vi "Teleop.vi"(10 "Match Info":T1={"Autonomous Elapsed Seconds"=0.0, "TeleOp Elapsed Seconds"=0.0, "Disabled Elapsed Seconds"=0.0, "Visited Autonomous"=FALSE, "Visited TeleOp"=FALSE, "Visited Disabled"=FALSE, "Autonomous Settings"={"Autonomous Style"=enum."Independent", "VI Refnum"=refnum}}, 11 "Call Context":T2) -> ()   [LabVIEW 2020]
doc: "This VI is called for each TeleOp packet received from the DS where the robot is not disabled. It is often used to read from the joysticks and update I/O or to update setpoints for timed control loops. It should complete and return within 20 milliseconds or it may miss DS packets."
uses:
  <vilib>/Rock Robotics/WPI/DriverStation/WPI_DriverStationDerivedRobotMode.ctl
  <vilib>/Rock Robotics/WPI/DriverStation/WPI_DriverStationMatch Info.ctl
  <vilib>/Rock Robotics/WPI/ThirdParty/Phoenix-LabVIEW/Motor Controller/Controls/CTRE_Phoenix_MotorControl_ControlMode.ctl
  <vilib>/Rock Robotics/WPI/Solenoid/WPI_SolenoidValue.ctl
  <vilib>/Rock Robotics/WPI/Utilities/WPI_GetSetVariantRefNum.vi
  <vilib>/Rock Robotics/Network Tables/NT Write Boolean Array.vi
  <vilib>/Rock Robotics/Network Tables/NT Write Numeric Array.vi
  <vilib>/Rock Robotics/Network Tables/NT Read Boolean.vi
  <vilib>/Rock Robotics/Network Tables/NT Read Number.vi
  Robot Global Data.vi
  <vilib>/Rock Robotics/WPI/ThirdParty/Phoenix-LabVIEW/Motor Controller/Get/CTRE_Phoenix_MotorController_GetSelectedSensorData.vi
  <vilib>/Rock Robotics/WPI/Solenoid/WPI_SolenoidSetEnum.vi
  <vilib>/Rock Robotics/WPI/ThirdParty/Phoenix-LabVIEW/Pigeon IMU/CTRE_PigeonIMU_GetAccumGyro.vi
panel:
  out "Left Motor Encoder":i32
  out "AccumGyro":cluster{"X":dbl, "Y":dbl, "Z":dbl}
  out "Intake Output":dbl
  out "Sample Slider 0":dbl(slide) scale=0.0..5.0
  out "Sample Boolean 1":bool
  out "Sample Boolean 0":bool
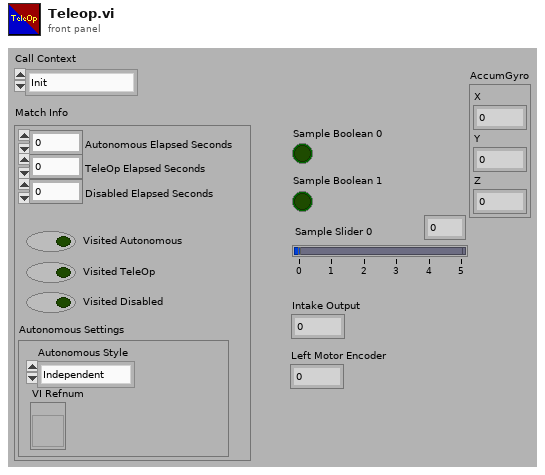
[diagram p1: front panel]
types:
  T1 = typedef "WPI_DriverStationMatch Info.ctl" = cluster{"Autonomous Elapsed Seconds":dbl, "TeleOp Elapsed Seconds":dbl, "Disabled Elapsed Seconds":dbl, "Visited Autonomous":bool, "Visited TeleOp":bool, "Visited Disabled":bool, "Autonomous Settings":cluster{"Autonomous Style":enum16{"Iterative", "Independent"}, "VI Refnum":refnum<vi>}}
  T2 = typedef "WPI_DriverStationDerivedRobotMode.ctl" = enum16{"Init", "Execute", "Stop"}
  T3 = typedef "WPI_SolenoidValue.ctl" = enum16{"Off", "On", "Forward", "Reverse"}
  T4 = typedef "CTRE_Phoenix_MotorControl_ControlMode.ctl" = u16
  T5 = typedef "WPI_JoystickDevRef.ctl" = cluster{"Device":T6}
  T6 = typedef "WPI_JoystickDeviceEnum.ctl" = enum16{"USB 0", "USB 1", "USB 2", "USB 3", "USB 4", "USB 5"}
  T7 = typedef "CTRE_PigeonIMU_DeviceRef.ctl" = cluster{"DeviceStatus":errorcluster, "Device Number":u8, "Type":T8, "Device ID":u32, "Handle":u64, "UsageFrame":u32, "Library Path":path}
  T8 = typedef "CTRE_PigeonIMU_ConnectionType.ctl" = u32
  T9 = typedef "WPI_MotorControlDeviceRef.ctl" = cluster{"DeviceStatus":errorcluster, "Type":T10, "PWM":cluster{"PWM Channel":T11, "DeadBand":T12}, "CAN":cluster{"Device Number":u8, "SetOutput VI Ref":variant, "GetOutput VI Ref":variant, "Enable VI Ref":variant, "Disable VI Ref":variant, "Data":variant}, "Invert":bool, "DIO PWM":cluster{"PWM \"Enable\" Channel":T11, "DIOChannel":T13, "PWM Rate":dbl}}
  T10 = typedef "WPI_MotorControlType.ctl" = enum16{"PWM", "CAN", "DIO PWM"}
  T11 = typedef "FPGA_DIOPWMChannel.ctl" = enum8{"PWM 0", "PWM 1", "PWM 2", "PWM 3", "PWM 4", "PWM 5", "PWM 6", "PWM 7", "PWM 8", "PWM 9", "PWM MXP 0", "PWM MXP 1", "PWM MXP 2", "PWM MXP 3", "PWM MXP 4", "PWM MXP 5", "PWM MXP 6", "PWM MXP 7", "PWM MXP 8", "PWM MXP 9", "Invalid"}
  T12 = typedef "WPI_PWMDeadband.ctl" = cluster{"Name":string, "maxPositivePwm":i32, "minPositivePwm":i32, "centerPwm":i32, "maxNegativePwm":i32, "minNegativePwm":i32, "angularRange":u16}
  T13 = typedef "FPGA_DIOChannel.ctl" = enum8{"DIO 0", "DIO 1", "DIO 2", "DIO 3", "DIO 4", "DIO 5", "DIO 6", "DIO 7", "DIO 8", "DIO 9", "DIO MXP 0", "DIO MXP 1", "DIO MXP 2", "DIO MXP 3", "DIO MXP 4", "DIO MXP 5", "DIO MXP 6", "DIO MXP 7", "DIO MXP 8", "DIO MXP 9", "DIO MXP 10", "DIO MXP 11", "DIO MXP 12", "DIO MXP 13", "DIO MXP 14", "DIO MXP 15", "SPI Port CS1", "SPI Port CS2", "SPI Port CS3", "SPI Port MISO", "SPI Port MOSI", "Invalid"}
  T14 = typedef "WPI_RobotDriveDevRef.ctl" = cluster{"DevStatus":errorcluster, "Motors[]":T9[], "Square Inputs":bool, "Max Output":dbl}
  T15 = typedef "WPI_SolenoidDevRef.ctl" = cluster{"DevStatus":errorcluster, "Pneumatics Control Module":u8, "Forward Solenoid Channel":T16, "Reverse Solenoid Channel":T16}
  T16 = typedef "WPI_SolenoidChannel.ctl" = enum8{"Solenoid 0", "Solenoid 1", "Solenoid 2", "Solenoid 3", "Solenoid 4", "Solenoid 5", "Solenoid 6", "Solenoid 7", "Solenoid 8", "Solenoid 9", "Solenoid 10", "Solenoid 11", "Solenoid 12", "Solenoid 13", "Solenoid 14", "Solenoid 15", "Invalid"}
  T17 = typedef "WPI_SwitchDevRef.ctl" = cluster{"DevStatus":errorcluster, "DIO Channel":T13, "CntIndex":T18, "Normally Closed":bool}
  T18 = typedef "FPGA_CounterCtrSystemIndex.ctl" = enum8{"Ctr 0", "Ctr 1", "Ctr 2", "Ctr 3", "Ctr 4", "Ctr 5", "Ctr 6", "Ctr 7", "Invalid"}
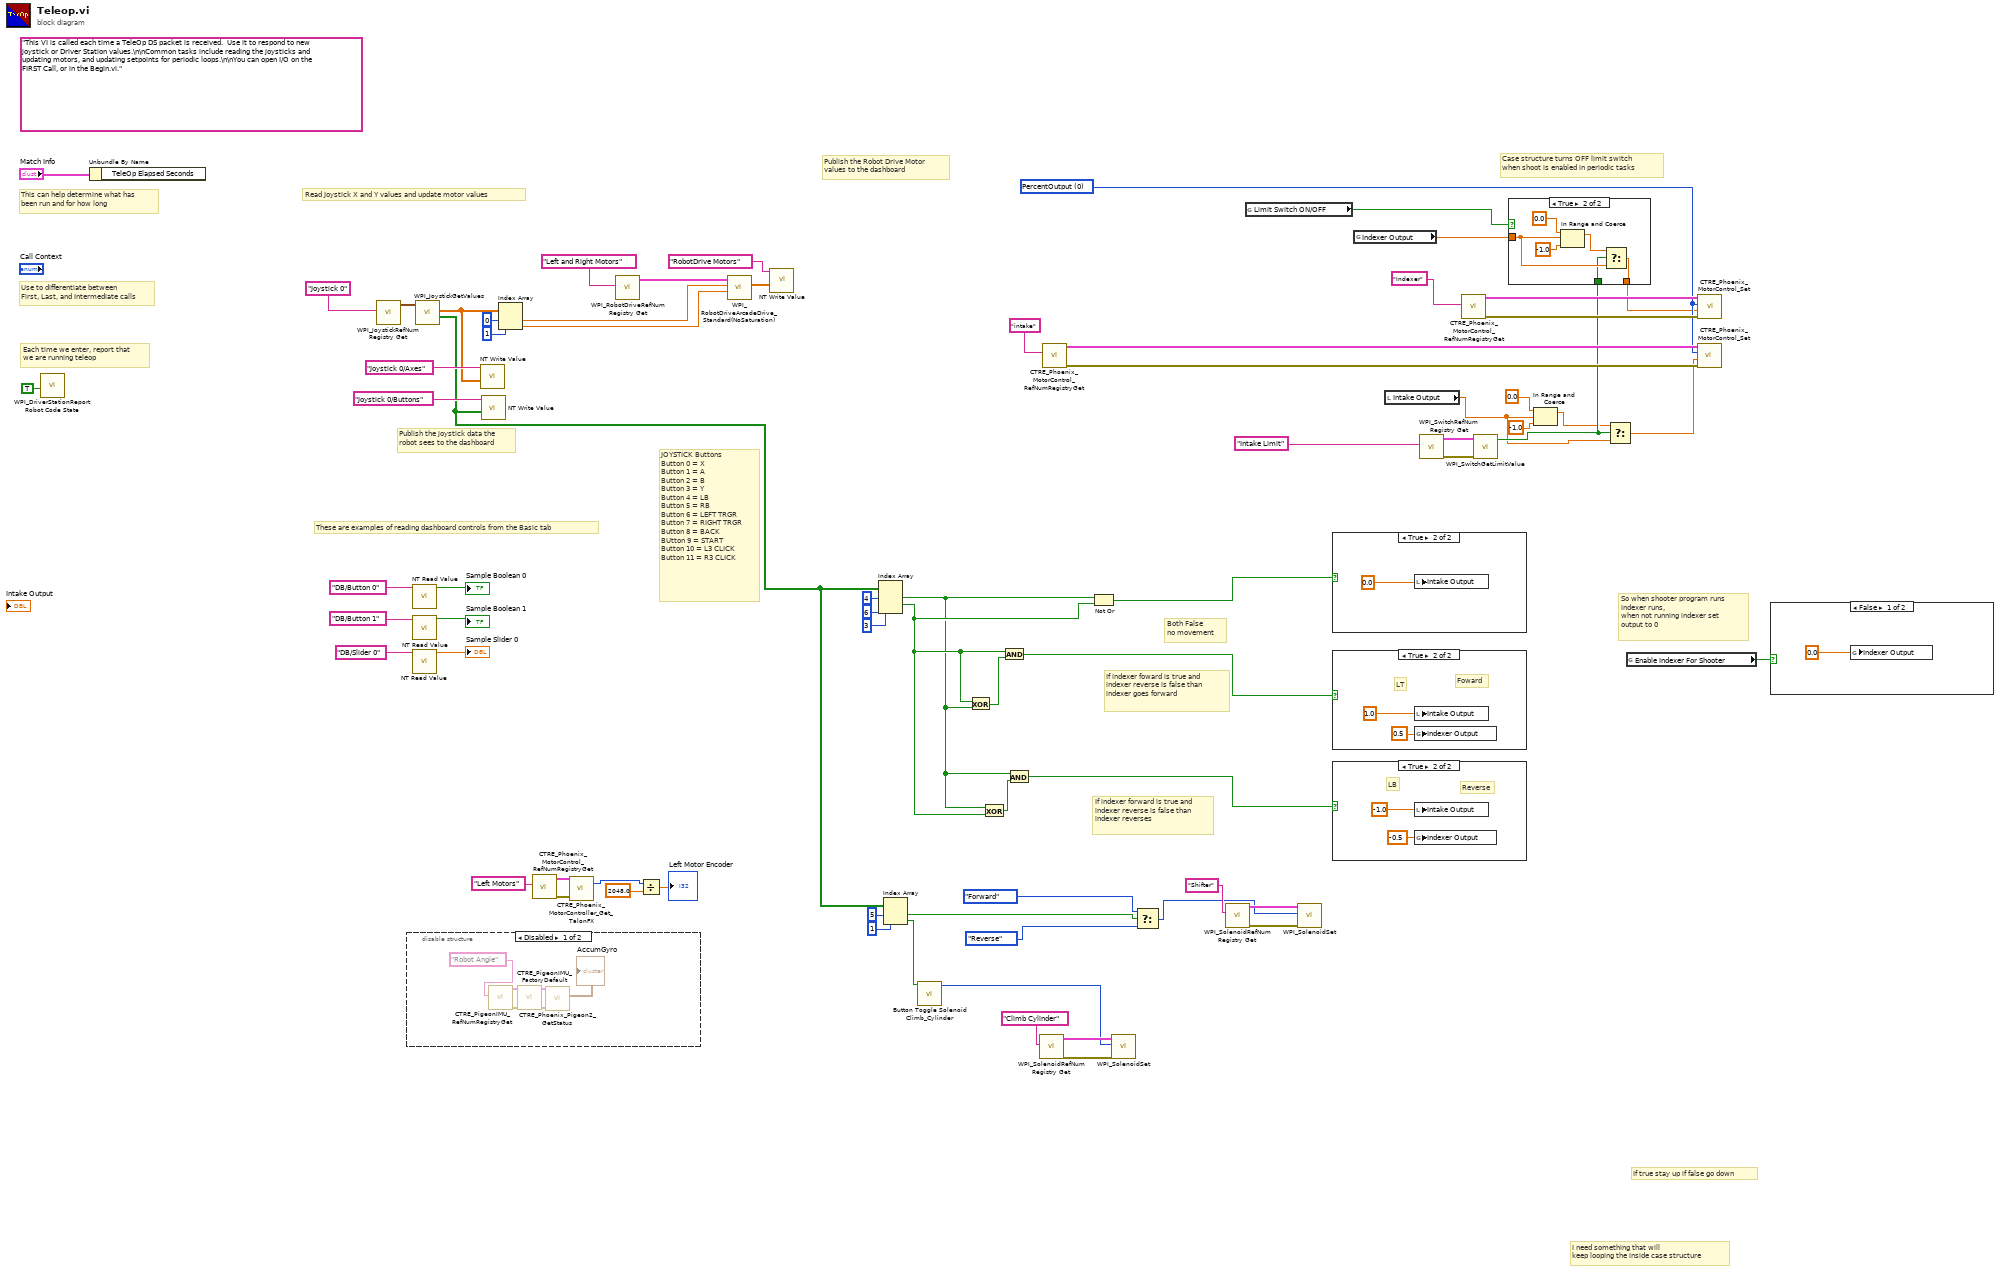
[diagram p0: block diagram]
diagram:
  w36 = T4 0 items=["PercentOutput"=0, "Position"=1, "Velocity"=2, "Current"=3, "Follower"=5, "MotionProfile"=6, "MotionMagic"=7, "MotionProfileArc"=10, "Disabled"=15] ("Control Mode")
  (unwired) "This VI is called each time a TeleOp DS packet is received.  Use it to respond to new joystick or Driver Station values.\n\nCommon tasks include reading the joysticks and updating motors, and updating setpoints for periodic loops.\n\nYou can open I/O on the FIRST Call, or in the Begin.vi."
  # "I need something that will\nkeep looping the inside case structure"
  # "If true stay up if false go down"
  # "So when shooter program runs\nindexer runs,\nwhen not running indexer set\noutput to 0"
  # "Case structure turns OFF limit switch\nwhen shoot is enabled in periodic tasks"
  # "If indexer foward is true and\nindexer reverse is false than \nindexer goes forward"
  # "Both False\nno movement"
  # "If indexer forward is true and\nindexer reverse is false than \nindexer reverses"
  # "JOYSTICK Buttons\nButton 0 = X\nButton 1 = A\nButton 2 = B\nButton 3 = Y\nButton 4 = LB \nButton 5 = RB\nButton 6 = LEFT TRGR \nButton 7 = RIGHT TRGR \nButton 8 = BACK\nBUtton 9 = START\nButton 10 = L3 CLICK\nButton 11 = R3 CLICK"
  # "These are examples of reading dashboard controls from the Basic tab"
  # "Publish the Robot Drive Motor\nvalues to the dashboard"
  # "Publish the joystick data the\nrobot sees to the dashboard"
  # "Each time we enter, report that\nwe are running teleop"
  # "Use to differentiate between\nFirst, Last, and Intermediate calls"
  # "This can help determine what has\nbeen run and for how long"
  # "Read Joystick X and Y values and update motor values"
  n1 = call <vilib>:"WPI_DriverStationReport Robot Code State.vi"("TeleOp"=TRUE ("Autonomous")) -> ()  [unwired: 10 in, 1 out]
  n2 = Unbundle By Name("Match Info") -> ()  [unwired: 1 out]
  n3 = call <vilib>:"WPI_JoystickRefNum Registry Get.vi"("refnum name"="Joystick 0") -> ("JoystickDevRef"=w70:T5)  [unwired: 1 in, 9 out]
  n4 = disable-structure shown="Disabled" {
    frame Disabled {
      n5 = call <vilib>:"CTRE_PigeonIMU_RefNumRegistryGet.vi"("refnum name"="Robot Angle") -> ("error out"=w74:errorcluster, "PigeonIMUDevRef"=w75:T7)  [unwired: 9 in]
      n6 = call <vilib>:"CTRE_PigeonIMU_FactoryDefault.vi"("error in"=w74, "PigeonIMUDevRef"=w75) -> ("error out"=w76:errorcluster, "PigeonIMUDevRef"=w77:T7)  [unwired: 8 in]
      n7 = call-poly <vilib>:"CTRE_Phoenix_Pigeon2_GetStatus.vi"("error in (no error)"=w76, "PigeonIMUDevRef"=w77) -> ("AccumGyro"=→"AccumGyro":cluster{"X":dbl, "Y":dbl, "Z":dbl})  [unwired: 7 in, 2 out]
    }
    frame Enabled {
    }
  }
  n8 = call-poly <vilib>:"NT Read Value.vi"("name"="DB/Button 0" ("refnum name")) -> ("value"=→"Sample Boolean 0":bool)  [unwired: 8 in, 2 out]
  n9 = call-poly <vilib>:"NT Read Value.vi"("name"="DB/Slider 0" ("refnum name")) -> ("value"=→"Sample Slider 0":dbl)  [unwired: 8 in, 2 out]
  n10 = call-poly <vilib>:"NT Read Value.vi"("name"="DB/Button 1" ("refnum name")) -> ("value"=→"Sample Boolean 1":bool)  [unwired: 8 in, 2 out]
  n11 = call <vilib>:"WPI_JoystickGetValues.vi"("JoystickDevRef"=w70) -> ("Buttons"=w15:bool[], "Axes"=w66:dbl[])  [unwired: 6 in, 3 out]
  n12 = call-poly <vilib>:"NT Write Value.vi"("value"=w66, "name"="Joystick 0/Axes" ("Name")) -> ()  [unwired: 9 in, 1 out]
  n13 = call-poly <vilib>:"NT Write Value.vi"("value"=w15, "name"="Joystick 0/Buttons" ("Name")) -> ()  [unwired: 9 in, 1 out]
  n14 = Index Array(array=w66, index #1=0 ("index"), index #2=1 ("index")) -> (element #1=w54:dbl, element #2=w53:dbl)
  n15 = call <vilib>:"CTRE_Phoenix_MotorControl_RefNumRegistryGet.vi"("refnum name"="Left Motors") -> ("error out"=w19:errorcluster, "PhoenixMotorControlDevRef"=w20:T9)  [unwired: 9 in]
  n16 = call-poly <vilib>:"CTRE_Phoenix_MotorController_Get_TalonFX.vi"("PhoenixMotorControlDevRef"=w20, "error in"=w19) -> ("Position (Raw Sensor Units)"=w16:i32)  [unwired: 10 in, 3 out]
  n17 = call <vilib>:"WPI_RobotDriveRefNum Registry Get.vi"("refnum name"="Left and Right Motors") -> ("RobotDriveDevRef"=w57:T14)  [unwired: 1 in, 9 out]
  n18 = Divide(x=w16, y=2048.0) -> (x/y=→"Left Motor Encoder":dbl)
  n19 = call <vilib>:"WPI_RobotDriveArcadeDrive_Standard(NoSaturation).vi"("Y axis value"=w53, "X axis value"=w54, "RobotDriveDevRef"=w57) -> ("Motor Values"=w56:dbl[])  [unwired: 1 in, 7 out]
  n20 = call-poly <vilib>:"NT Write Value.vi"("value"=w56, "name"="RobotDrive Motors" ("Name")) -> ()  [unwired: 9 in, 1 out]
  n21 = Index Array(array=w15, index #1=4 ("index"), index #2=6 ("index"), index #3=3 ("index")) -> (element #1=w42:bool, element #2=w43:bool)  [unwired: 1 out]
  n22 = Index Array(array=w15, index #1=5 ("index"), index #2=1 ("index")) -> (element #1=w3:bool, element #2=w1:bool)
  n23 = call "Button Toggle Solenoid Climb_Cylinder.vi"("Button A"=w1) -> ("Climb_Cylinder_Value"=w2:T3)  [unwired: 10 in]
  n24 = Exclusive Or(1:w42, 2:w43) -> (0:w50:bool)
  n25 = Exclusive Or(1:w43, 2:w42) -> (0:w49:bool)
  n26 = And(x=w43, y=w50) -> (x .and. y?=w48:bool)
  n27 = And(x=w42, y=w49) -> (x .and. y?=w47:bool)
  n28 = call <vilib>:"WPI_SolenoidRefNum Registry Get.vi"("refnum name"="Climb Cylinder") -> ("error out"=w6:errorcluster, "SolenoidDevRef"=w7:T15)  [unwired: 9 in]
  n29 = call <vilib>:"CTRE_Phoenix_MotorControl_RefNumRegistryGet.vi"("refnum name"="intake") -> ("error out"=w40:errorcluster, "PhoenixMotorControlDevRef"=w41:T9)  [unwired: 9 in]
  n30 = Not Or(1:w43, 2:w42) -> (0:w44:bool)
  n31 = call-poly <vilib>:"WPI_SolenoidSet.vi"("error in (no error)"=w6, "Value"=w2, "SolenoidDevRef"=w7) -> ()  [unwired: 7 in, 2 out]
  n32 = Select(t=WPI_SolenoidValue."Forward" ("Value"), s=w3, f=WPI_SolenoidValue."Reverse" ("Value")) -> (s? t:f=w10:T3)
  n33 = call <vilib>:"WPI_SolenoidRefNum Registry Get.vi"("refnum name"="Shifter") -> ("error out"=w12:errorcluster, "SolenoidDevRef"=w11:T15)  [unwired: 9 in]
  n34 = global read "Robot Global Data.vi" "Limit Switch ON/OFF"() -> (w24:bool)
  n35 = call-poly <vilib>:"WPI_SolenoidSet.vi"("error in (no error)"=w12, "Value"=w10, "SolenoidDevRef"=w11) -> ()  [unwired: 7 in, 2 out]
  n36 = case shown="True" w44 {
    frame False {
    }
    frame True {
      n37 = local write "Intake Output"(0.0) -> ()
    }
  }
  n38 = case shown="True" w48 {
    frame False {
    }
    frame True {
      # "Foward"
      # "LT"
      n39 = local write "Intake Output"(1.0) -> ()
      n40 = global write "Robot Global Data.vi" "Indexer Output"(0.5 ("Indexer Output")) -> ()
    }
  }
  n41 = case shown="True" w47 {
    frame False {
    }
    frame True {
      # "Reverse"
      # "LB"
      n42 = local write "Intake Output"(-1.0) -> ()
      n43 = global write "Robot Global Data.vi" "Indexer Output"(-0.5 ("Indexer Output")) -> ()
    }
  }
  n44 = global read "Robot Global Data.vi" "Indexer Output"() -> (w25:dbl)
  n45 = local read "Intake Output"() -> (w34:dbl)
  n46 = call <vilib>:"WPI_SwitchRefNum Registry Get.vi"("refnum name"="Intake Limit") -> ("error out"=w33:errorcluster, "SwitchDevRef"=w30:T17)  [unwired: 9 in]
  n47 = call <vilib>:"CTRE_Phoenix_MotorControl_RefNumRegistryGet.vi"("refnum name"="Indexer") -> ("error out"=w37:errorcluster, "PhoenixMotorControlDevRef"=w38:T9)  [unwired: 9 in]
  n48 = call <vilib>:"WPI_SwitchGetLimitValue.vi"("error in (no error)"=w33, "SwitchDevRef"=w30) -> ("Switch Pressed"=w35:bool)  [unwired: 7 in, 2 out]
  n49 = case shown="True" w24 {
    tunnel: w35 -> [_ w85]
    tunnel: [w84 w86] -> w26
    tunnel: w25 -> [w84 w87]
    frame False {
    }
    frame True {
      n50 = In Range and Coerce(upper limit=0.0, x=w87, lower limit=-1.0) -> (coerced(x)=w90:dbl)  [unwired: 1 out]
      n51 = Select(t=w90, s=w85, f=w87) -> (s? t:f=w86:dbl)
    }
  }
  n52 = In Range and Coerce(upper limit=0.0, x=w34, lower limit=-1.0) -> (coerced(x)=w31:dbl)  [unwired: 1 out]
  n53 = Select(t=w31, s=w35, f=w34) -> (s? t:f=w27:dbl)
  n54 = global read "Robot Global Data.vi" "Enable Indexer For Shooter"() -> (w22:bool)
  n55 = call <vilib>:"CTRE_Phoenix_MotorControl_Set.vi"("error in (no error)"=w40, "Output"=w27, "Control Mode"=w36, "PhoenixMotorControlDevRef"=w41) -> ()  [unwired: 6 in, 2 out]
  n56 = call <vilib>:"CTRE_Phoenix_MotorControl_Set.vi"("error in (no error)"=w37, "Output"=w26, "Control Mode"=w36, "PhoenixMotorControlDevRef"=w38) -> ()  [unwired: 6 in, 2 out]
  n57 = case shown="False" w22 {
    frame False {
      n58 = global write "Robot Global Data.vi" "Indexer Output"(0.0) -> ()
    }
    frame True {
    }
  }
